vi "PicoScope6000SetDataBuffersSingle.vi"(5 "enabled array":i16[](array[numeric]), 7 "Buffer and Transfer Settings":T2 {"Down-Sample Mode" items=["RAW none", "None", "Aggregate", "Decimate", "Average"]; "Down Sample Ratio" step=1; "Samples" format="%_6p"}, 8 "error in (no error)":errorcluster, 9 "waveform":i32, 10 "Data Pointers In":T1, 11 "handle in":i16) -> (0 "error out":errorcluster, 3 "handle out":i16)   [LabVIEW 2009]
doc: "Calls SetDataBuffers, and assigns Pico buffers"
uses:
  ps6000.dll
  shared/PicoBuffers.ctl
  shared/Buffer and Transfer Settings.ctl
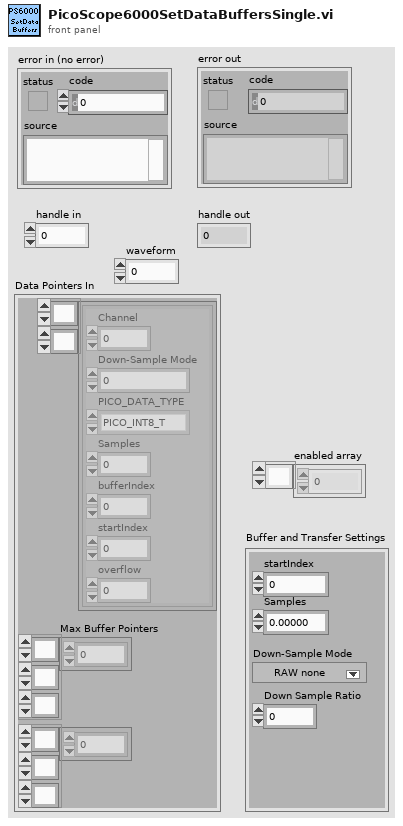
[diagram p1: front panel]
types:
  T1 = typedef "PicoBuffers.ctl" = cluster{"Max Buffer Pointers":u64[][][], "Min Buffer Pointers":u64[][][], "StreamingDataInfo":cluster{"Channel":u32, "Down-Sample Mode":u32, "PICO_DATA_TYPE":enum32{"PICO_INT8_T", "PICO_INT16_T", "PICO_INT32_T", "PICO_UINT32_T", "PICO_INT64_T", ""}, "Samples":i32, "bufferIndex":u64, "startIndex":i32, "overflow":i16}[][]}
  T2 = typedef "Buffer and Transfer Settings.ctl" = cluster{"startIndex":u64, "Samples":u64, "Down Sample Ratio":u64, "Down-Sample Mode":u32}
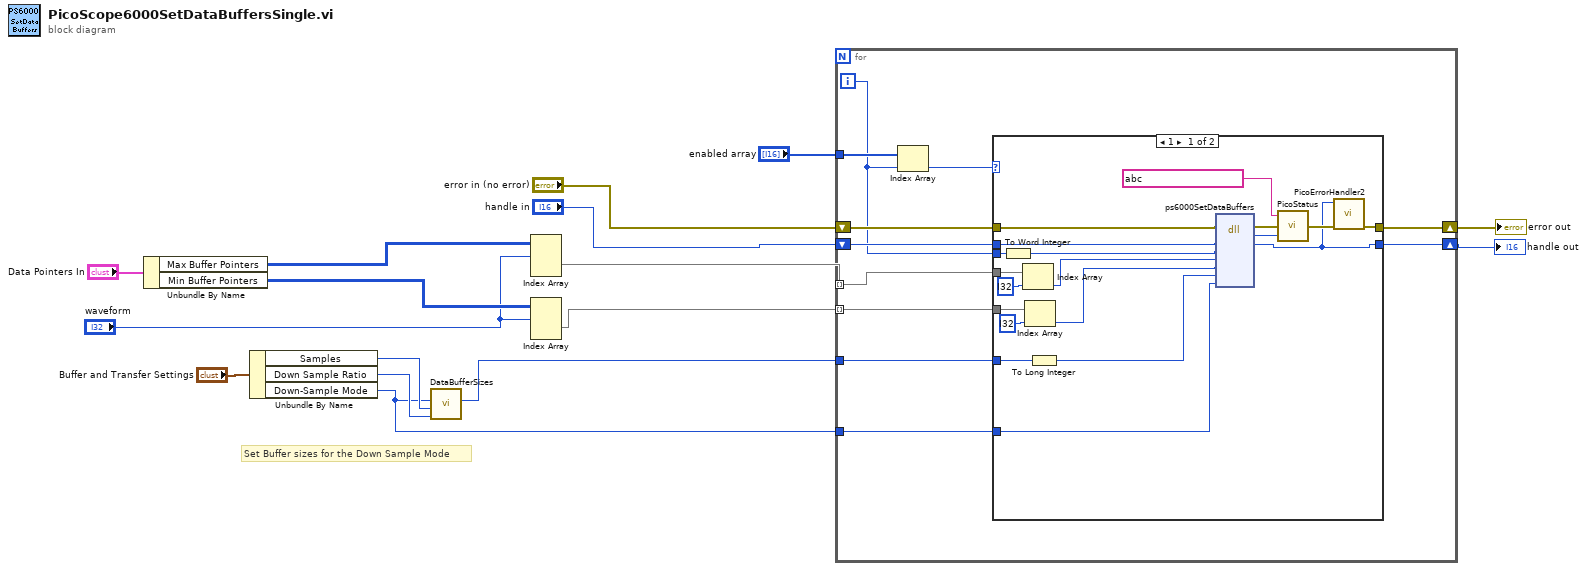
[diagram p0: block diagram]
diagram:
  # "Set Buffer sizes for the Down Sample Mode"
  n1 = Unbundle By Name("Data Pointers In") -> ("Max Buffer Pointers"=w5:u64[][][], "Min Buffer Pointers"=w2:u64[][][])
  n2 = Unbundle By Name("Buffer and Transfer Settings") -> ("Samples"=w8:u64, "Down Sample Ratio"=w9:u64, "Down-Sample Mode"=w7:u32)
  n3 = call "DataBufferSizes.vi"("Down Sample Ratio"=w9, "Number of Samples"=w8, "Down-Sample Mode"=w7) -> ("Max Buffer Size"=w10:i32)  [unwired: 7 in, 1 out]
  n4 = Index Array(array=w5, index (dim 0)="waveform") -> (element=w4:u64[][])  [unwired: 2 in]
  n5 = Index Array(array=w2, index (dim 0)="waveform") -> (element=w3:u64[][])  [unwired: 2 in]
  n6 = for {
    tunnel: w7 -> [w27]
    tunnel: w10 -> [w22]
    tunnel: "enabled array" -> [w24]
    tunnel: w4 -> [w21] mode=indexing
    shift-right: [w20] -> w15
    shift-left: "error in (no error)" -> [w26]
    tunnel: w3 -> [w19] mode=indexing
    shift-right: [w18] -> w14
    shift-left: "handle in" -> [w25]
    i -> [w17]
    n7 = Index Array(array=w24, index=w17) -> (element=w23:i16)
    n8 = case shown="1" w23 {
      tunnel: w17 -> [w43 _]
      tunnel: w26 -> [w38 w48]
      tunnel: w25 -> [w37 w47]
      tunnel: w27 -> [w28 _]
      tunnel: [w45 w48] -> w20
      tunnel: [w29 w47] -> w18
      tunnel: w22 -> [w44 _]
      tunnel: w21 -> [w41 _]
      tunnel: w19 -> [w39 _]
      frame #0 {
        n9 = To Word Integer(number=w43) -> (16bit integer=w36:i16)
        n10 = Index Array(array=w41, index=i32 ?) -> (element=w35:u64)
        n11 = Index Array(array=w39, index=i32 ?) -> (element=w34:u64)
        n12 = To Long Integer(number=w44) -> (32bit integer=w33:i32)
        n13 = dll-call lib="ps6000.dll" fn="ps6000SetDataBuffers" ("ps3000.dll:_ps3000_open_unit@0")(error in=w38, "handle"=w37, "channel"=w36, "bufferMax"=w35, "bufferMin"=w34, "bufferLth"=w33, "downSampleRatioMode"=w28) -> (error out=w32:errorcluster, "PICO_STATUS"=w30:u32, "handle"=w29:i16)  [unwired: 7 in, 1 out]
        n14 = call "PicoStatus.vi"("PICO STATUS"=w30, "error in"=w32, "source"=string ?) -> ("error out"=w31:errorcluster)
        n15 = call "PicoErrorHandler2.vi"("error in (no error)"=w31, "handle In"=w29) -> ("error out"=w45:errorcluster)  [unwired: 9 in]
      }
      frame #1 {
      }
    }
  }
  "error out" <- w15
  "handle out" <- w14
